vi "Grafica Convencional.vi"() -> ()   [LabVIEW 2017]
uses:
  <vilib>/MakerHub/LINX/Public/Peripherals/Digital/Digital Write 1 Chan.vi
  <vilib>/MakerHub/LINX/Private/Local IO/LinxI2cWrite.vi
  <vilib>/MakerHub/LINX/Public/Utilities/Check Channel.vi
  <vilib>/MakerHub/LINX/Public/Peripherals/Digital/Digital Write N Chans.vi
  <vilib>/MakerHub/LINX/Private/Local IO/LinxDigitalWrite.vi
  <vilib>/MakerHub/LINX/Public/Utilities/Open Serial.vi
  <vilib>/MakerHub/LINX/Private/Utilties/Generate Error.vi
  <vilib>/MakerHub/LINX/LMH-LINX.lvlib
panel:
  out "Valor recibido":string
  out "Generador convencional":i32(graph)
  out "Valor graficado":i32
  in  "Prueba":bool
  out "Bytes recibidos por i2c":u8[](array[numeric])
  in  "Dirección I2C generador convencional":u8
  out "Tarjeta de adquisición de datos":string
  in  "Puerto serial de la tarjeta":refnum<visa-resource-name>="N/A"
  in  "stop":bool
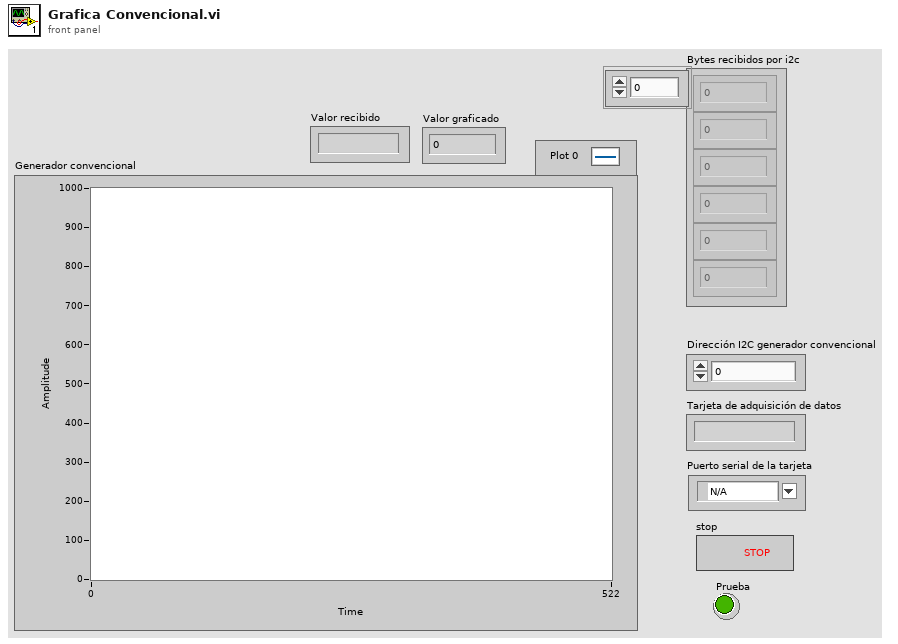
[diagram p1: front panel]
types:
  T1 = typedef "LMH-LINX.lvlib/LINX Ref.ctl" = cluster{"IO":T2, "Interface":T3, "LINX Device Config":T4}
  T2 = typedef "LMH-LINX.lvlib/Platform.ctl" = enum16{"Remote", "Local"}
  T3 = typedef "LMH-LINX.lvlib/Interface.ctl" = enum16{"Serial", "TCP"}
  T4 = typedef "LMH-LINX.lvlib/Device.lvlib/LINX Device Config.ctl" = cluster{"Interface":T3, "COM Port":refnum<visa-resource-name>, "TCP Configuration":T5, "Device Family":u8, "Device ID":u8, "Device Name":string, "TCP Ref":refnum<k5>, "Channels":T6}
  T5 = typedef "LMH-LINX.lvlib/Device.lvlib/TCP Config.ctl" = cluster{"IP Address":string, "Port":u16}
  T6 = typedef "LMH-LINX.lvlib/Channels.ctl" = cluster{"DI":u8[], "DO":u8[], "AI":u8[], "AO":u8[], "PWM":u8[], "QE":u8[], "UART":u8[], "I2C 2":u8[], "SPI":u8[], "CAN":u8[], "Servo":u8[], "AI Ref (V)":dbl, "AI Resolution (Bits)":u8, "AO Ref (V)":dbl, "AO Resolution (Bits)":u8}
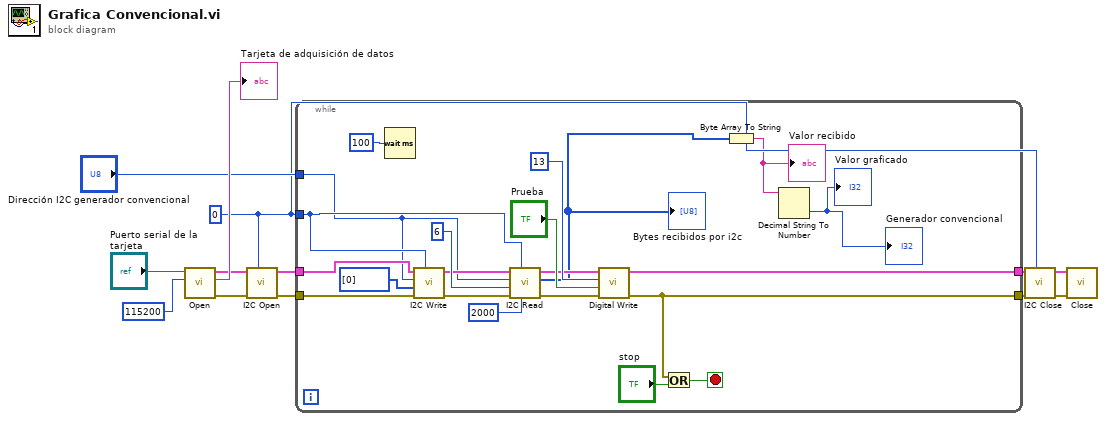
[diagram p0: block diagram]
diagram:
  w3 = u8 0 ("I2C Channel (0)")
  n1 = call-poly <vilib>:"Open.vi"("Baud Rate Override"=u32 115200, "Serial Port"="Puerto serial de la tarjeta") -> ("Error Out"=w9:errorcluster, "Device Name"=→"Tarjeta de adquisición de datos":string, "LINX Resource"=w8:T1)  [unwired: 7 in]
  n2 = call <vilib>:"I2C Open.vi"("I2C Channel (0)"=w3, "Error In"=w9, "LINX Resource"=w8) -> ("Error Out"=w7:errorcluster, "LINX Resource"=w6:T1)  [unwired: 7 in]
  n3 = while {
    tunnel: "Dirección I2C generador convencional" -> [w18]
    tunnel: w7 -> [w20]
    tunnel: w6 -> [w21]
    tunnel: w3 -> [w19]
    tunnel: [w30] -> w2
    tunnel: [w27] -> w1
    stop <- w28 stop-if-true
    n4 = Wait (ms)(milliseconds to wait=u32 100) -> ()  [unwired: 1 out]
    n5 = call <vilib>:"I2C Write.vi"("I2C Channel"=w19, "Error In"=w20, "Data"=u8[] [0], "I2C Slave Address (0)"=w18, "LINX Resource"=w21) -> ("Error Out"=w22:errorcluster, "LINX Resource"=w23:T1)  [unwired: 5 in]
    n6 = call <vilib>:"I2C Read.vi"("Timeout (1000 ms)"=u16 2000, "I2C Channel"=w19, "Error In"=w22, "Bytes To Read"=u8 6, "I2C Slave Address (0)"=w18, "LINX Resource"=w23) -> ("Error Out"=w32:errorcluster, "Data"=w16:u8[], "LINX Resource"=w31:T1)  [unwired: 3 in]
    "Bytes recibidos por i2c" <- w16
    n7 = call-poly <vilib>:"Digital Write.vi"("Error In"=w32, "Output Value"="Prueba", "DO Channel"=u8 13, "LINX Resource"=w31) -> ("Error Out"=w27:errorcluster, "LINX Resource"=w30:T1)  [unwired: 6 in]
    n8 = Or(x=w27, y="stop") -> (x .or. y?=w28:bool)
    n9 = Byte Array To String(unsigned byte array=w16) -> (string=w15:string)
    "Valor recibido" <- w15
    n10 = Decimal String To Number(string=w15) -> (number=→"Valor graficado" →"Generador convencional":i32)  [unwired: 2 in, 1 out]
  }
  n11 = call <vilib>:"I2C Close.vi"("I2C Channel (0)"=w3, "Error In"=w1, "LINX Resource"=w2) -> ("Error Out"=w5:errorcluster, "LINX Resource"=w4:T1)  [unwired: 7 in]
  n12 = call <vilib>:"Close.vi"("Error In"=w5, "LINX Resource"=w4) -> ()  [unwired: 9 in, 1 out]
